vi "U32ToU16.vi"(5 "Number":u32) -> (1 "Unsigned 16-bit integer":u16, 2 "Overflow?":bool, 3 "Exact conversion?":bool)   [LabVIEW 2017, in "GPOverflow.lvlib"]
doc: "Converts <B>Number</B> to U16 keeping track of numeric overflow and exactness of conversion.\n\n<B>Exact conversion?</B> will be True only if a conversion back into the original data type of <B>Number</B> will yield the exact same number, i.e. no precision was lost during the conversion.\n\n<B>Overflow?</B> will be True if positive or negative overflow occurred. The numeric output will saturate in case of overflow.\n\nThis VI is inlined.\n\nSteen Schmidt\nGPower\n6/3 2013"
uses:
  GPOverflow.lvlib
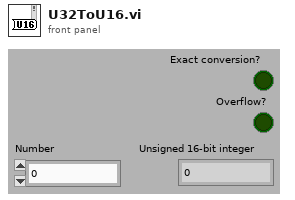
[diagram p1: front panel]
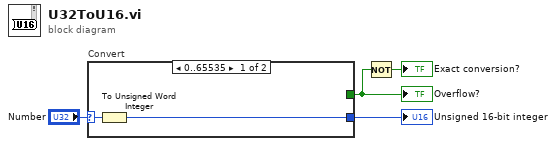
[diagram p0: block diagram]
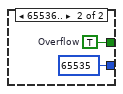
[diagram p2: hidden frame]
diagram:
  n1 = case "Convert" shown="0..65535" "Number" {
    selector: "Number" -> [w6 _]
    tunnel: [w5 u16 65535] -> w3
    tunnel: [_ w7] -> w2
    frame 0..65535 {
      n2 = To Unsigned Word Integer(number=w6) -> (unsigned 16bit integer=w5:u16)
    }
    frame 65536.. {
      w7 = TRUE  # Overflow
    }
  }
  "Unsigned 16-bit integer" <- w3
  "Overflow?" <- w2
  n3 = Not(x=w2) -> (.not. x?=→"Exact conversion?":bool)
